vi "Actor Core.vi"(8 "error in":errorcluster, 11 "NHMFL Synthesizer in":refnum<class "NHMFL Synthesizer.lvclass">) -> (0 "error out":errorcluster, 3 "Actor out":refnum<class "Actor.lvclass">)   [LabVIEW 2016, in "NHMFL Synthesizer.lvclass"]
doc: "(<B>Filename</B>: Actor Framework.lvlib:Actor.lvclass:Actor Core.vi)\n\nReceives messages to the actor, reacts to them, and initiates any error handling that may shut the actor down.\n\nDescendant classes may override this VI to append parallel tasks for the actor to complete while it handles messages. Overrides use the Call Parent Method node."
uses:
  NHMFL Synthesizer.lvclass
  D:/github/Measure_core/Da Base/Da Base.lvclass
  D:/Program Files/National Instruments/LabVIEW 2016/vi.lib/ActorFramework/Actor/Actor.lvclass
  <vilib>/ActorFramework/Actor/Actor.lvclass
  NHMFL_Core/Libraries/NI-DAQ/NHMFL Synthesizer/Actual Settings.ctl
  NHMFL_Core/Libraries/NI-DAQ/NHMFL Synthesizer/NHMFL Synthesizer Configuration.ctl
  Measure_core/Da Base/Da Base.lvclass/Da Base.ctl
  <vilib>/ActorFramework/Actor/Actor.lvclass/Actor.ctl
  <vilib>/ActorFramework/Message Enqueuer/Message Enqueuer.lvclass/Message Enqueuer.ctl
  Measure_core/da Base/Read stop event.vi
  <vilib>/ActorFramework/Message Enqueuer/Init from Existing Queue.vi
  <vilib>/ActorFramework/Message Enqueuer/Enqueue.vi
  NHMFL Synthesizer Messages/Program Synth Msg/Program Synth Msg.lvclass
  D:/Program Files/National Instruments/LabVIEW 2016/vi.lib/ActorFramework/Message/Message.lvclass
  <vilib>/ActorFramework/Message Priority Queue/Priority Enqueue.vi
  Measure_core/Process Object/Process Object.lvclass
  <vilib>/ActorFramework/Message Enqueuer/Message Enqueuer.lvclass
panel:
  out "Name":string
  in  "Program":bool
  in  "Configuration":T1={"DAQmx Device"="", "Variable amplitude frequency"=256000.0, "Fixed amplitude frequency"=nan, "Amplitude"=2.1, "Clock multiplier"=75, "Cannel names (variable F)"=[], "Cannel names (fixed F)"=[], "Group"="p"} {"Amplitude" format="%#_6pV"; "Fixed amplitude frequency" format="%#_6pHz"; "Variable amplitude frequency" format="%#_6pHz"}
  out "Actual settings":T2 {"Clock" format="%_20p"; "F2" format="%_20p"; "F1" format="%_20p"; "Clock/F2" format="%_20g"; "Clock/F1" format="%_20g"}
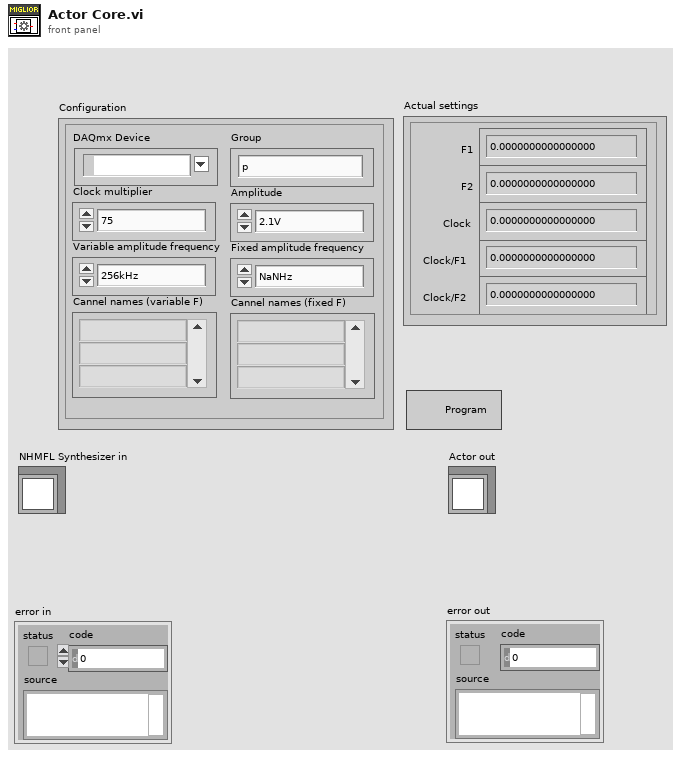
[diagram p1: front panel]
types:
  T1 = typedef "NHMFL Synthesizer Configuration.ctl" = cluster{"DAQmx Device":tag, "Variable amplitude frequency":dbl, "Fixed amplitude frequency":dbl, "Amplitude":dbl, "Clock multiplier":i32, "Cannel names (variable F)":string[], "Cannel names (fixed F)":string[], "Group":string}
  T2 = typedef "Actual Settings.ctl" = cluster{"Clock/F1":ext, "Clock/F2":ext, "F1":ext, "F2":ext, "Clock":ext}
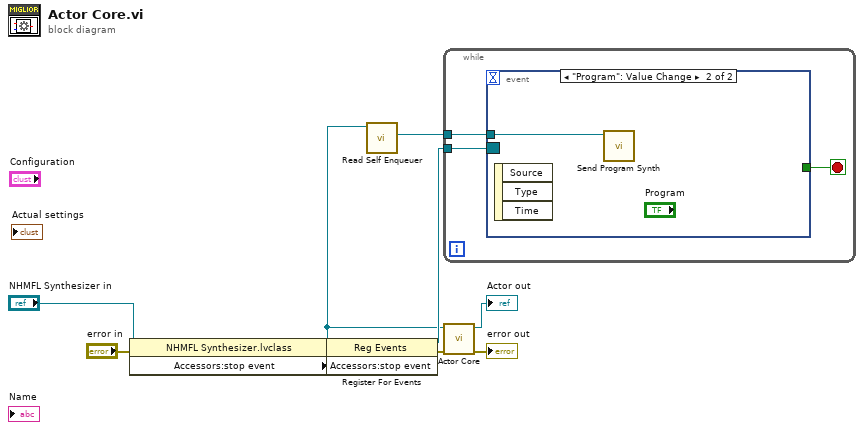
[diagram p0: block diagram]
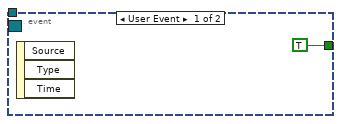
[diagram p2: hidden frame]
diagram:
  n1 = property class="NHMFL Synthesizer.lvclass"(reference="NHMFL Synthesizer in", error in="error in") -> (reference out=w2:refnum<class "NHMFL Synthesizer.lvclass">, error out=w8:errorcluster, "Accessors:stop event"=w7:refnum<user-event>)
  n2 = register-events(error in=w8, w7) -> (reference out=w6:refnum<event-registration>, error out=w1:errorcluster)  [unwired: 1 in]
  n3 = call <vilib>:"Read Self Enqueuer.vi"("Actor"=w2) -> ("Self Enqueuer"=w5:refnum<class "Message Enqueuer.lvclass">)  [unwired: 10 in]
  n4 = while {
    tunnel: w6 -> [w13]
    tunnel: w5 -> [w11]
    stop <- w12 stop-if-true
    n5 = event shown="[1] \"Program\": Value Change" {
      selector: w13 -> [_ _]
      dyn-events: _ -> [_ _]
      timeout: _ -> [_ _]
      tunnel: [TRUE _] -> w12
      tunnel: w11 -> [_ w15]
      event User Event {
        n6 = event-data() -> ()  [unwired: 1 in, 3 out]
      }
      event "Program": Value Change {
        n7 = event-data() -> ()  [unwired: 1 in, 3 out]
        n8 = call "Send Program Synth.vi"("Message Enqueuer"=w15) -> ()  [unwired: 9 in, 2 out]
      }
    }
  }
  n9 = call-parent "Actor Core.vi"("error in"=w1, "Measure Object in"=w2) -> ("error out"=→"error out":errorcluster, "Actor out"=→"Actor out":refnum<class "Actor.lvclass">)  [unwired: 8 in]
